vi "replaceEasyXMLDefaultName.vi"(8 "error in":errorcluster, 10 "desiredName":string, 11 "easyXMLStringWithDefaultNames":string) -> (0 "error out":errorcluster, 3 "xmlString":string)   [LabVIEW 2016, in "UnitsAndXML.lvlib"]
uses:
  <userlib>/Common/UnitsAndXML/UnitsAndXML.lvlib
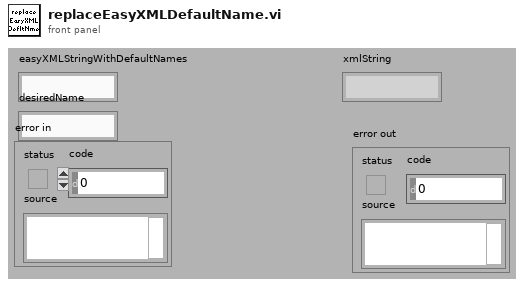
[diagram p1: front panel]
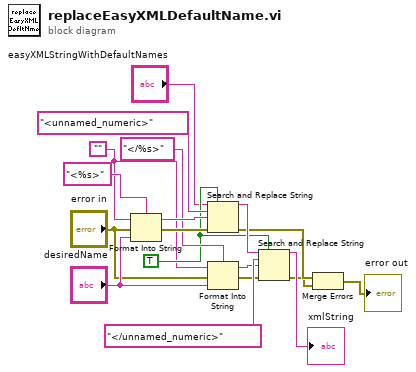
[diagram p0: block diagram]
diagram:
  w1 = ""
  w10 = TRUE ("replace all? (F)")
  n1 = Format Into String(format string="<%s>" ("search string"), initial string=w1, error in="error in", "desiredName") -> (resulting string=w17:string, error out=w18:errorcluster)
  n2 = Search and Replace String(replace all?=w10, input string="easyXMLStringWithDefaultNames", search string="<unnamed_numeric>", replace string=w17, error in=w18) -> (result string=w11:string, error out=w4:errorcluster)  [unwired: 3 in, 2 out]
  n3 = Format Into String(format string="</%s>" ("search string"), initial string=w1, error in="error in", "desiredName") -> (resulting string=w6:string, error out=w12:errorcluster)
  n4 = Search and Replace String(replace all?=w10, input string=w11, search string="</unnamed_numeric>", replace string=w6, error in=w12) -> (result string=→"xmlString":string, error out=w3:errorcluster)  [unwired: 3 in, 2 out]
  n5 = Merge Errors(w4, w3) -> (→"error out":errorcluster)
